vi "Write Strings.vi"(8 "error in (no error)":errorcluster, 10 "Strings":refnum<class "Abs_Value.lvclass">[](array[class]), 11 "Concatenate_STR in":refnum<class "Concatenate_STR.lvclass">) -> (0 "error out":errorcluster, 3 "Concatenate_STR out":refnum<class "Concatenate_STR.lvclass">)   [LabVIEW 2021, in "Concatenate_STR.lvclass"]
uses:
  Concatenate_STR.lvclass
  Abs_Types/Value/Abs_Value.lvclass
  Concatenate_STR.lvclass/Concatenate_STR.ctl
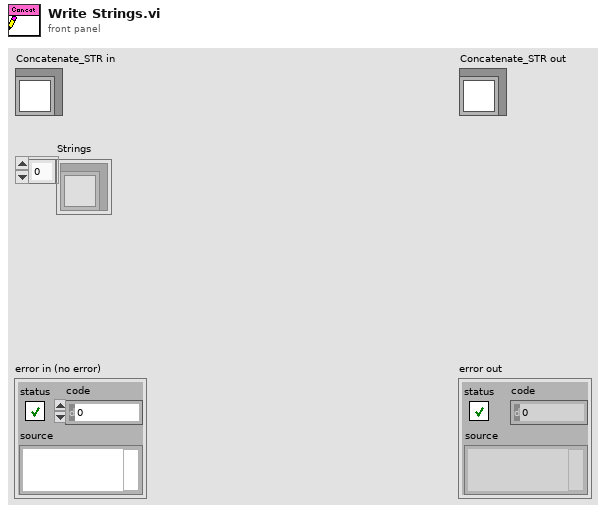
[diagram p1: front panel]
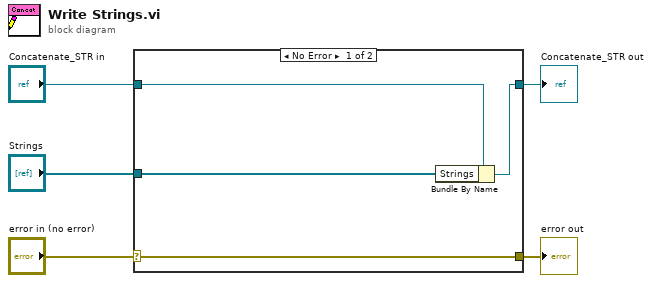
[diagram p0: block diagram]
diagram:
  n1 = case shown="No Error" "error in (no error)" {
    selector: "error in (no error)" -> [w9 w10]
    tunnel: [w9 w10] -> w4
    tunnel: [w7 w11] -> w2
    tunnel: "Concatenate_STR in" -> [w8 w11]
    tunnel: "Strings" -> [w6 _]
    frame No Error {
      n2 = Bundle By Name(cluster=w8, "Strings"=w6) -> (w7:refnum<class "Concatenate_STR.lvclass">)
    }
    frame Error {
    }
  }
  "error out" <- w4
  "Concatenate_STR out" <- w2
